vi "Set Gear Ratio.vi"(6 "subpanel to main command event":T1, 8 "error in (no error)":errorcluster, 10 "gear ratio":dbl, 11 "steering frame ref in":refnum<data-value>) -> (0 "error out":errorcluster, 3 "steering frame ref out":refnum<data-value>)   [LabVIEW 2017, in "NI_Robotics_Configure Steering Frame.lvlib" / "Mecanum Frame Subpanel.lvlib"]
uses:
  <vilib>/robotics/Dialog/Configure Steering Frame/Mecanum Frame Subpanel/Mecanum Frame Subpanel.lvlib
  <vilib>/robotics/Steering/Mecanum Steering Frame/NI_Robotics_Mecanum Steering Frame.lvclass
  c:/Program Files (x86)/National Instruments/LabVIEW 2017/vi.lib/robotics/Steering/Steering Frame/NI_Robotics_Steering Frame.lvclass
  <vilib>/robotics/Dialog/Configure Steering Frame/Subpanel to Main Command Event.ctl
  <vilib>/robotics/Dialog/Configure Steering Frame/Subpanel to Main Command.ctl
  <vilib>/robotics/Dialog/Configure Steering Frame/Generate Subpanel to Main Event.vi
  <vilib>/robotics/Steering/Steering Frame/NI_Robotics_Steering Frame.lvclass
  <vilib>/robotics/Dialog/Configure Steering Frame/NI_Robotics_Configure Steering Frame.lvlib
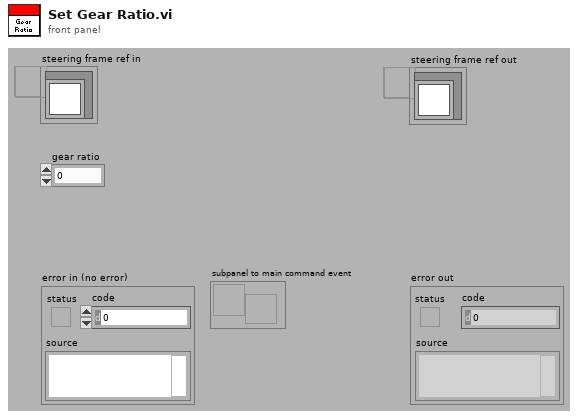
[diagram p1: front panel]
types:
  T1 = typedef "NI_Robotics_Configure Steering Frame.lvlib/Subpanel to Main Command Event.ctl" = refnum<user-event>
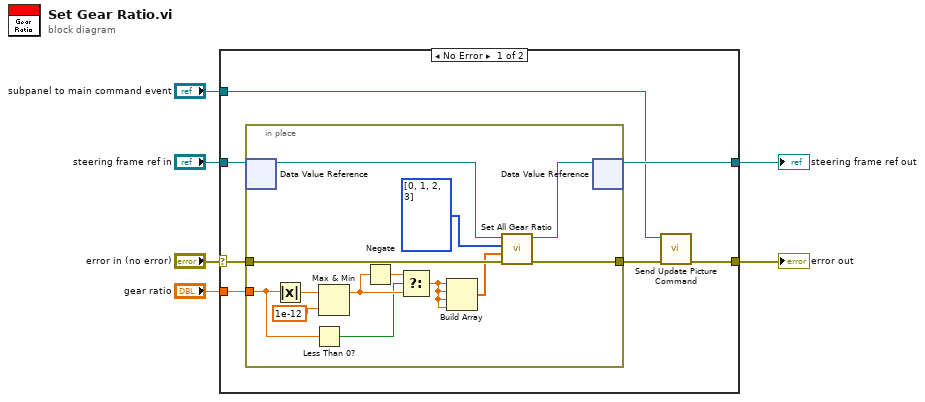
[diagram p0: block diagram]
diagram:
  n1 = case shown="No Error" "error in (no error)" {
    selector: "error in (no error)" -> [w12 w27]
    tunnel: "steering frame ref in" -> [w13 w28]
    tunnel: [w10 w28] -> w4
    tunnel: [w7 w27] -> w3
    tunnel: "subpanel to main command event" -> [w9 _]
    tunnel: "gear ratio" -> [w11 _]
    frame No Error {
      n2 = in-place {
        in-place-border: w12 -> [w24]
        in-place-border: w11 -> [w15]
        in-place-border: [w23] -> w8
        n3 = in-place-dvr #1(w13) -> (w26:refnum<class "NI_Robotics_Mecanum Steering Frame.lvclass">)  [unwired: 1 out]
        n4 = Absolute Value(x=w15) -> (abs(x)=w16:dbl)
        n5 = Less Than 0?(x=w15) -> (x < 0?=w18:bool)
        n6 = Max & Min(x=w16, y=1e-12) -> (max(x,y)=w19:dbl)  [unwired: 1 out]
        n7 = Negate(x=w19) -> (-x=w20:dbl)
        n8 = Select(t=w20, s=w18, f=w19) -> (s? t:f=w14:dbl)
        n9 = Build Array(w14, w14, w14, w14) -> (w21:dbl[])
        n10 = call <vilib>:"Set All Gear Ratio.vi"("error in (no error)"=w24, "gear ratio"=w21, "wheel indexes"=i32[] [0, 1, 2, 3], "steering frame in"=w26) -> ("error out"=w23:errorcluster, "steering frame out"=w25:refnum<class "NI_Robotics_Mecanum Steering Frame.lvclass">)  [unwired: 5 in, 1 out]
        n11 = in-place-dvr #1(w25) -> (w10:refnum<data-value>)  [unwired: 1 out]
      }
      n12 = call <vilib>:"Send Update Picture Command.vi"("error in (no error)"=w8, "subpanel to main command event"=w9) -> ("error out"=w7:errorcluster)  [unwired: 9 in]
    }
    frame Error {
    }
  }
  "steering frame ref out" <- w4
  "error out" <- w3
